vi "First Step.vi"(8 "error in (no error)":errorcluster, 11 "Magnetic Field.lvclass in":refnum<class "Magnetic Field.lvclass">) -> (0 "error out":errorcluster, 2 "Current Position":dbl, 3 "Magnetic Field.lvclass out":refnum<class "Magnetic Field.lvclass">)   [LabVIEW 2017, in "Magnetic Field.lvclass"]
uses:
  Magnetic Field.lvclass
  Instruments/Magnet/Power Supply/Power Supply.lvclass
  C:/LabVIEW-programs-dev/Instruments/Utility Classes/Scannable/Scannable.lvclass
  Scanner/Scanner.lvclass
panel:
  out "persis?":bool caption="Persistent"
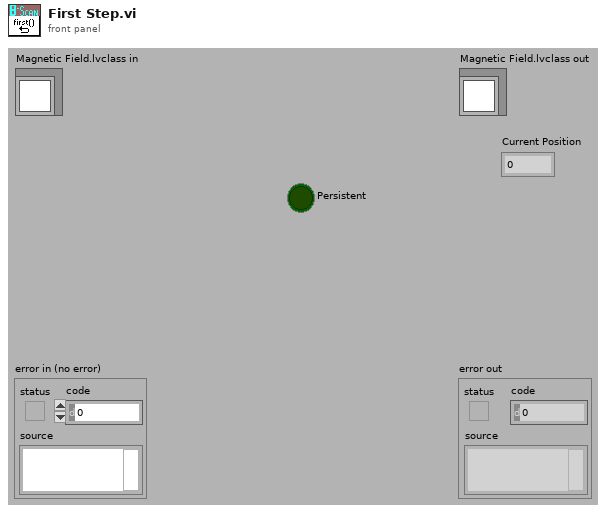
[diagram p1: front panel]
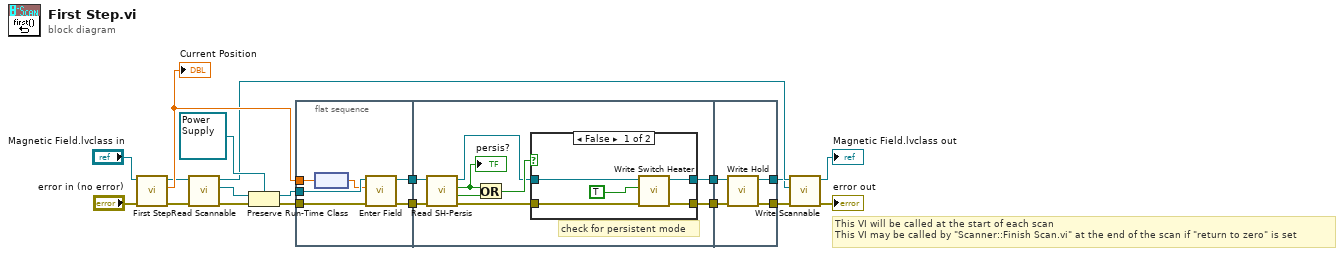
[diagram p0: block diagram]
diagram:
  # "This VI will be called at the start of each scan\nThis VI may be called by \"Scanner::Finish Scan.vi\" at the end of the scan if \"return to zero\" is set"
  n1 = call-parent "First Step.vi"("error in (no error)"="error in (no error)", "Scanner.lvclass in"="Magnetic Field.lvclass in") -> ("error out"=w2:errorcluster, "Current Position"=w17:dbl, "Scanner.lvclass out"=w13:refnum<class "Magnetic Field.lvclass">)  [unwired: 7 out]
  "Current Position" <- w17
  n2 = call-dynamic "Read Scannable.vi"("error in (no error)"=w2, "Scanner.lvclass in"=w13) -> ("error out"=w16:errorcluster, "Scannable.lvclass"=w15:refnum<class "Scannable.lvclass">, "Scanner.lvclass out"=w11:refnum<class "Magnetic Field.lvclass">)  [unwired: 7 in]
  n3 = Preserve Run-Time Class(object in=w15, error in=w16, 2:refnum<class "Power Supply.lvclass"> refnum ("Power Supply in")) -> (object out=w10:refnum<class "Power Supply.lvclass">, error out=w3:errorcluster)
  n4 = flat-sequence {
    tunnel: w17 -> [w25]
    tunnel: w10 -> [w24]
    tunnel: [w23] -> w9
    tunnel: [w22] -> w4
    tunnel: w3 -> [w21]
    tunnel: w9 -> [w31]
    tunnel: [w29] -> w8
    tunnel: [w28] -> w5
    tunnel: w4 -> [w26]
    tunnel: w8 -> [w45]
    tunnel: [w44] -> w7
    tunnel: [w43] -> w6
    tunnel: w5 -> [w42]
    frame #0 {
      n5 = node(w25) -> (w20:dbl[unit])
      n6 = call-dynamic "Enter Field.vi"("error in (no error)"=w21, "Target field"=w20, "Power Supply in"=w24) -> ("error out"=w22:errorcluster, "Power Supply out"=w23:refnum<class "Power Supply.lvclass">)  [unwired: 7 in]
    }
    frame #1 {
      # "check for persistent mode"
      n7 = call-dynamic "Read SH-Persis.vi"("error in (no error)"=w26, "Power Supply in"=w31) -> ("error out"=w27:errorcluster, "SHon?"=w33:bool, "pers?"=w32:bool, "Power Supply out"=w30:refnum<class "Power Supply.lvclass">)  [unwired: 4 in, 2 out]
      "persis?" <- w32
      n8 = Or(x=w32, y=w33) -> (x .or. y?=w34:bool)
      n9 = case shown="False" w34 {
        tunnel: w30 -> [w39 w41]
        tunnel: [w38 w41] -> w29
        tunnel: [w37 w40] -> w28
        tunnel: w27 -> [w36 w40]
        frame False {
          n10 = call-dynamic "Write Switch Heater.vi"("error in (no error)"=w36, "Turn SH On?"=TRUE, "Power Supply in"=w39) -> ("error out"=w37:errorcluster, "Power Supply out"=w38:refnum<class "Power Supply.lvclass">)  [unwired: 7 in]
        }
        frame True {
        }
      }
    }
    frame #2 {
      n11 = call-dynamic "Write Hold.vi"("error in (no error)"=w42, "Power Supply in"=w45) -> ("error out"=w43:errorcluster, "Power Supply out"=w44:refnum<class "Power Supply.lvclass">)  [unwired: 8 in]
    }
  }
  n12 = call-dynamic "Write Scannable.vi"("error in (no error)"=w6, "Scannable.lvclass"=w7, "Scanner.lvclass in"=w11) -> ("error out"=→"error out":errorcluster, "Scanner.lvclass out"=→"Magnetic Field.lvclass out":refnum<class "Magnetic Field.lvclass">)  [unwired: 7 in]
